vi "SWERVE_ODOM_ABS_ACQUIRE.vi"(4 "visionRobotPose":T1={"TRANSLATION"={"X"=0.0, "Y"=0.0}, "ROTATION"={"VALUE"=0.0, "COS"=1.0, "SIN"=0.0}} {"ROTATION"."SIN" format="%13.4f"; "ROTATION"."COS" format="%13.4f"; "ROTATION"."VALUE" format="%13.4f"; "TRANSLATION"."Y" format="%14.3f"; "TRANSLATION"."X" format="%14.3f"}, 5 "Game Started":bool, 6 "Add Vision Meas":bool, 7 "InitialPose":T1={"TRANSLATION"={"X"=0.0, "Y"=0.0}, "ROTATION"={"VALUE"=0.0, "COS"=1.0, "SIN"=0.0}} {"ROTATION"."SIN" format="%13.4f"; "ROTATION"."COS" format="%13.4f"; "ROTATION"."VALUE" format="%13.4f"; "TRANSLATION"."Y" format="%14.3f"; "TRANSLATION"."X" format="%14.3f"}, 8 "VisionLatency_sec":dbl=0.2 format="%#_13g", 9 "in Swerve Module Positions":T7[](array[typedef]) {"Angle"."SIN" format="%13.4f"; "Angle"."COS" format="%13.4f"; "Angle"."VALUE" format="%13.4f"}, 10 "Gyro_Heading_Rad":dbl, 11 "in SWERVE_DRIVE_KINEMATICS":T4 {"SavedModuleStates"."Angle"."SIN" format="%13.4f"; "SavedModuleStates"."Angle"."COS" format="%13.4f"; "SavedModuleStates"."Angle"."VALUE" format="%13.4f"; "PrevCoR"."Y" format="%14.3f"; "PrevCoR"."X" format="%14.3f"; "Modules"."Y" format="%14.3f"; "Modules"."X" format="%14.3f"}) -> (0 "POSE_EST_POSE":T1={"TRANSLATION"={"X"=0.0, "Y"=0.0}, "ROTATION"={"VALUE"=0.0, "COS"=1.0, "SIN"=0.0}} {"ROTATION"."SIN" format="%13.4f"; "ROTATION"."COS" format="%13.4f"; "ROTATION"."VALUE" format="%13.4f"; "TRANSLATION"."Y" format="%14.3f"; "TRANSLATION"."X" format="%14.3f"}, 2 "ODOM_POSE":T1={"TRANSLATION"={"X"=0.0, "Y"=0.0}, "ROTATION"={"VALUE"=0.0, "COS"=1.0, "SIN"=0.0}} {"ROTATION"."SIN" format="%13.4f"; "ROTATION"."COS" format="%13.4f"; "ROTATION"."VALUE" format="%13.4f"; "TRANSLATION"."Y" format="%14.3f"; "TRANSLATION"."X" format="%14.3f"})   [LabVIEW 2023]
uses:
  <vilib>/Rock Robotics/WPI/ThirdParty/JAS_Junk/TrajLib/TypeDef/SWERVE_DRIVE_MODULE_POSITION.ctl
  <vilib>/Rock Robotics/WPI/ThirdParty/JAS_Junk/TrajLib/TypeDef/ROTATION2D.ctl
  <vilib>/Rock Robotics/WPI/ThirdParty/JAS_Junk/TrajLib/TypeDef/SWERVE_DRIVE_KINEMATICS.ctl
  <vilib>/Analysis/Matrix/Datatypes/RealMatrix.ctl
  <vilib>/Rock Robotics/WPI/ThirdParty/JAS_Junk/TrajLib/TypeDef/TRANSLATION2D.ctl
  <vilib>/Rock Robotics/WPI/ThirdParty/JAS_Junk/TrajLib/TypeDef/SWERVE_DRIVE_MODULE_STATE.ctl
  <vilib>/Rock Robotics/WPI/ThirdParty/JAS_Junk/TrajLib/TypeDef/POSE2D.ctl
  <vilib>/Rock Robotics/WPI/ThirdParty/JAS_Junk/TrajLib/VI/Util_GetTime_U32.vi
  <vilib>/Rock Robotics/WPI/ThirdParty/JAS_Junk/TrajLib/Rotation2d_Plus.vi
  <vilib>/Rock Robotics/WPI/ThirdParty/JAS_Junk/TrajLib/Twist2d_Create.vi
  <vilib>/Rock Robotics/WPI/ThirdParty/JAS_Junk/TrajLib/Rotation2d_Minus.vi
  <vilib>/Rock Robotics/WPI/ThirdParty/JAS_Junk/TrajLib/Pose2d_getTranslation.vi
  <vilib>/Rock Robotics/WPI/ThirdParty/JAS_Junk/TrajLib/Pose2d_New_TRRO.vi
  <vilib>/Rock Robotics/WPI/ThirdParty/JAS_Junk/TrajLib/VI/SwerveModulePosition_Get.vi
  <vilib>/Rock Robotics/WPI/ThirdParty/JAS_Junk/TrajLib/VI/SwerveModulePosition_New.vi
  <vilib>/Rock Robotics/WPI/ThirdParty/JAS_Junk/TrajLib/Twist2d_GetAll.vi
  <vilib>/Rock Robotics/WPI/ThirdParty/JAS_Junk/TrajLib/Pose2d_getRotation.vi
  <vilib>/Rock Robotics/WPI/ThirdParty/JAS_Junk/TrajLib/VI/TimeInterpVariant_Clear.vi
  <vilib>/Rock Robotics/WPI/ThirdParty/JAS_Junk/TrajLib/Rotation2d_RotateBy.vi
  <vilib>/Rock Robotics/WPI/ThirdParty/JAS_Junk/TrajLib/Rotation2d_UnaryMinus.vi
  <vilib>/Rock Robotics/WPI/ThirdParty/JAS_Junk/TrajLib/Rotation2d_CreateXY.vi
  <vilib>/Rock Robotics/WPI/ThirdParty/JAS_Junk/TrajLib/Util_CalcDist.vi
  <vilib>/Rock Robotics/SystemInterfaces/Utilities/FPGA_UtilitiesRead LocalTime.vi
  <vilib>/Rock Robotics/WPI/ThirdParty/JAS_Junk/TrajLib/VI/Util_GetTime_U64.vi
  <vilib>/Rock Robotics/WPI/ThirdParty/JAS_Junk/TrajLib/VI/SwerveKinematics_ToTwist2dX.vi
  <vilib>/Rock Robotics/WPI/ThirdParty/JAS_Junk/TrajLib/Pose2d_Exp.vi
  <vilib>/Rock Robotics/WPI/ThirdParty/JAS_Junk/TrajLib/Trajectory_Library.lvlib
  <vilib>/Analysis/Matrix/NI_Matrix.lvlib
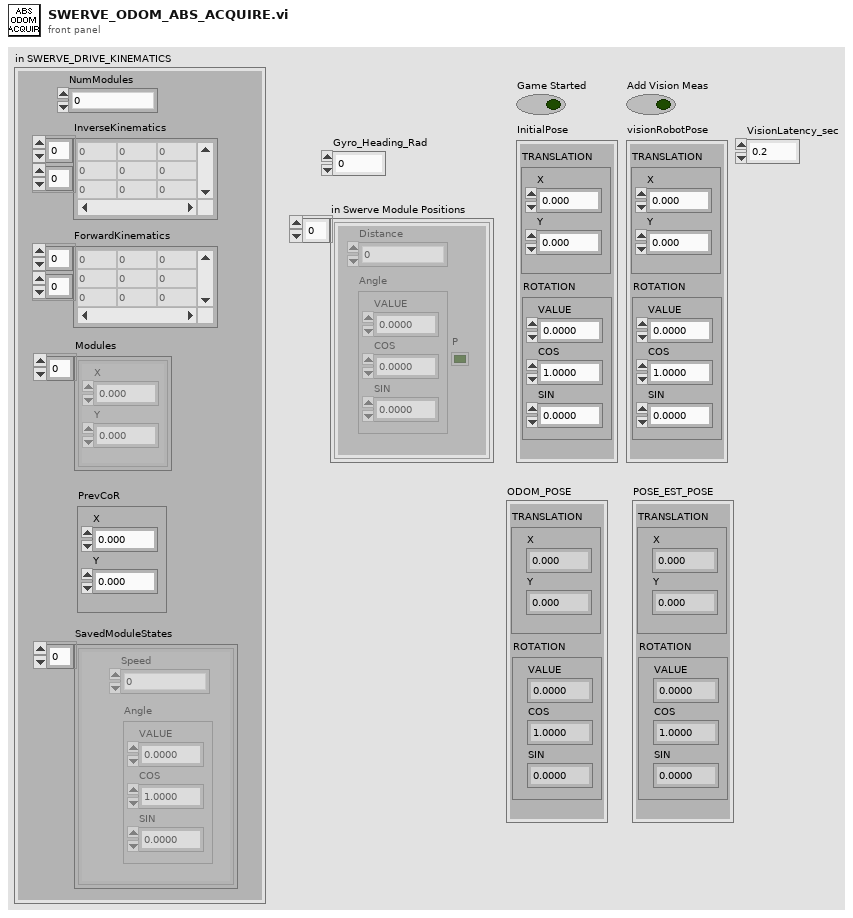
[diagram p1: front panel]
types:
  T1 = typedef "Trajectory_Library.lvlib/POSE2D.ctl" = cluster{"TRANSLATION":T2, "ROTATION":T3}
  T2 = typedef "Trajectory_Library.lvlib/TRANSLATION2D.ctl" = cluster{"X":dbl, "Y":dbl}
  T3 = typedef "Trajectory_Library.lvlib/ROTATION2D.ctl" = cluster{"VALUE":dbl, "COS":dbl, "SIN":dbl}
  T4 = typedef "Trajectory_Library.lvlib/SWERVE_DRIVE_KINEMATICS.ctl" = cluster{"NumModules":i32, "InverseKinematics":T5, "ForwardKinematics":T5, "Modules":T2[], "PrevCoR":T2, "SavedModuleStates":T6[]}
  T5 = typedef "NI_Matrix.lvlib/RealMatrix.ctl" = dbl[][]
  T6 = typedef "Trajectory_Library.lvlib/SWERVE_DRIVE_MODULE_STATE.ctl" = cluster{"Speed":dbl, "Angle":T3}
  T7 = typedef "Trajectory_Library.lvlib/SWERVE_DRIVE_MODULE_POSITION.ctl" = cluster{"Distance":dbl, "Angle":T3, "P":bool}
  T8 = typedef "Trajectory_Library.lvlib/SWERVE_DRIVE_POSE_EST2.ctl" = cluster{"M_Vision_K":T5, "m_nominal_dT":dbl, "m_PrevTime_Sec":dbl, "Pose_Buffer":T9, "Swerve_Drive_Kinematics":T4, "Swerve_Drive_Odom":T10, "M_Q":T5, "NumModules":i32}
  T9 = typedef "Trajectory_Library.lvlib/TIME_INTERPOLATABLE_VARIANT.ctl" = cluster{"TimeStamps":dbl[], "DataArray":variant[], "Min_TimeStamp":dbl, "Max_TimeStamp":dbl, "ItemCount":i32, "MaxBufferTime":dbl}
  T10 = typedef "Trajectory_Library.lvlib/SWERVE_DRIVE_ODOMETRY.ctl" = cluster{"POSE":T1, "GyroOffset":T3, "PreviousAngle":T3, "PrevModulePositions":T7[], "NumModules":i32}
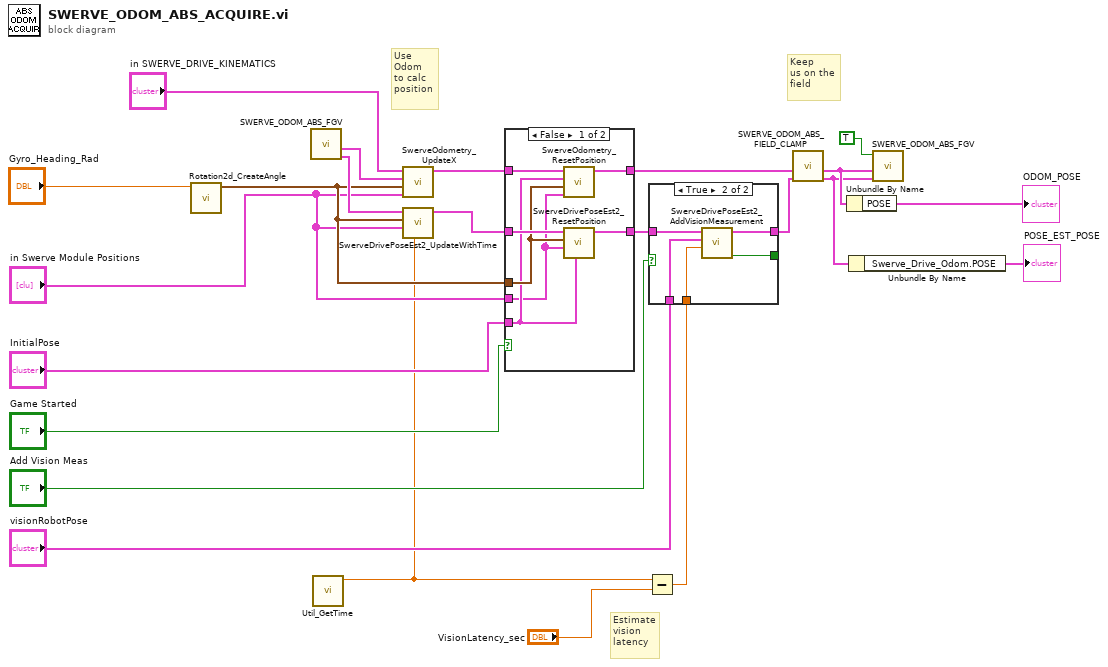
[diagram p0: block diagram]
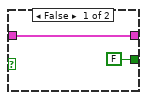
[diagram p3: hidden frame]
diagram:
  # "Estimate\nvision \nlatency"
  # "Keep\nus on the\nfield"
  # "Use\nOdom\nto calc\nposition"
  n1 = call <vilib>:"Rotation2d_CreateAngle.vi"("Angle"="Gyro_Heading_Rad") -> ("ROTATION"=w14:T3)  [unwired: 10 in]
  n2 = call "SWERVE_ODOM_ABS_FGV.vi"() -> ("out SWERVE_DRIVE_POSE_EST2"=w19:T8, "out SWERVE_DRIVE_ODOMETRY"=w22:T10)  [unwired: 10 in]
  n3 = call <vilib>:"Util_GetTime.vi"() -> ("FPGA_Time_Seconds"=w2:dbl)  [unwired: 9 in, 2 out]
  n4 = call <vilib>:"SwerveOdometry_UpdateX.vi"("module Positions"="in Swerve Module Positions", "gyroAngle"=w14, "in SWERVE_DRIVE_ODOMETRY"=w22, "SWERVE_DRIVE_KINEMATICS"="in SWERVE_DRIVE_KINEMATICS") -> ("out SWERVE_DRIVE_ODOMETRY"=w18:T10)  [unwired: 5 in, 2 out]
  n5 = call <vilib>:"SwerveDrivePoseEst2_UpdateWithTime.vi"("CurrentTimeSeconds"=w2, "module Positions"="in Swerve Module Positions", "GyroAngle"=w14, "in SwerveDrivePoseEst2"=w19) -> ("Out SwerveDrivePoseEst2"=w17:T8)  [unwired: 5 in, 2 out]
  n6 = case shown="False" "Game Started" {
    tunnel: w17 -> [w30 w32]
    tunnel: w14 -> [w26 _]
    tunnel: "in Swerve Module Positions" -> [w24 _]
    tunnel: "InitialPose" -> [w25 _]
    tunnel: [w29 w32] -> w16
    tunnel: w18 -> [w28 w31]
    tunnel: [w27 w31] -> w9
    frame False {
      n7 = call <vilib>:"SwerveOdometry_ResetPosition.vi"("Module Positions"=w24, "gyroAngle"=w26, "Pose"=w25, "in SWERVE_DRIVE_ODOMETRY"=w28) -> ("out SWERVE_DRIVE_ODOMETRY"=w27:T10)  [unwired: 6 in, 1 out]
      n8 = call <vilib>:"SwerveDrivePoseEst2_ResetPosition.vi"("Pose"=w25, "Module Positions"=w24, "Gyro"=w26, "in SwerveDrivePoseEst2"=w30) -> ("Out SwerveDrivePoseEst2"=w29:T8)  [unwired: 7 in]
    }
    frame True {
    }
  }
  n9 = Subtract(x=w2, y="VisionLatency_sec") -> (x-y=w1:dbl)
  n10 = case shown="True" "Add Vision Meas" {
    tunnel: w16 -> [w34 w39]
    tunnel: [w34 w38] -> w8
    tunnel: [FALSE ("Error") w37] -> _
    tunnel: "visionRobotPose" -> [_ w36]
    tunnel: w1 -> [_ w35]
    frame False {
    }
    frame True {
      n11 = call <vilib>:"SwerveDrivePoseEst2_AddVisionMeasurement.vi"("TImeStamp_Seconds"=w35, "visionRobotPose"=w36, "in SwerveDrivePoseEst2"=w39) -> ("Error"=w37:bool, "Out SwerveDrivePoseEst2"=w38:T8)  [unwired: 7 in]
    }
  }
  n12 = call "SWERVE_ODOM_ABS_FIELD_CLAMP.vi"("in SWERVE_DRIVE_POSE_EST2"=w8, "in SWERVE_DRIVE_ODOMETRY"=w9) -> ("out SWERVE_DRIVE_POSE_EST2"=w6:T8, "out SWERVE_DRIVE_ODOMETRY"=w7:T10)  [unwired: 8 in]
  n13 = Unbundle By Name(w7) -> ("POSE"=→"ODOM_POSE":T1)
  n14 = Unbundle By Name(w6) -> ("Swerve_Drive_Odom.POSE"=→"POSE_EST_POSE":T1)
  n15 = call "SWERVE_ODOM_ABS_FGV.vi"("in SWERVE_DRIVE_POSE_EST2"=w6, "in SWERVE_DRIVE_ODOMETRY"=w7, "WRITE"=TRUE) -> ()  [unwired: 7 in, 2 out]
